vi "Initialize Signal Array.vi"(6 "error out":errorcluster, 9 "signal list":refnum<k21>[](array[refnum])) -> (0 "error out":errorcluster, 3 "Array":dbl[](array[numeric]))   [LabVIEW 2015]
uses:
  <vilib>/xnet/xnet.llb/XNET Database Open (Signal).vi
  <vilib>/xnet/xnet.llb/XNET Database Close (Signal).vi
  <resource>/objmgr/xnet.rc
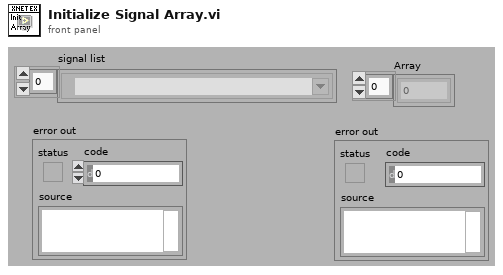
[diagram p1: front panel]
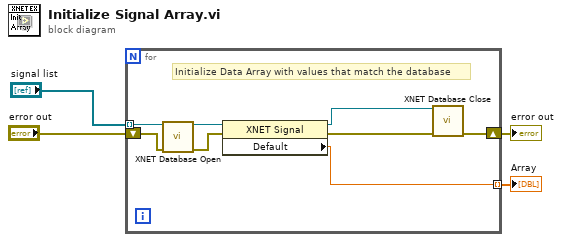
[diagram p0: block diagram]
diagram:
  n1 = for {
    tunnel: "signal list" -> [w12] mode=indexing
    shift-right: [w7] -> w3
    shift-left: "error out" -> [w11]
    tunnel: [w5] -> w1 mode=indexing
    # "Initialize Data Array with values that match the database"
    n2 = call-poly <vilib>:"XNET Database Open.vi"("signal in"=w12, "error in (no error)"=w11) -> ("signal out"=w10:refnum<k21>, "error out"=w9:errorcluster)  [unwired: 12 in]
    n3 = property class="XNET Signal"(reference=w10, error in=w9) -> (reference out=w6:refnum<k21>, error out=w8:errorcluster, "Default"=w5:dbl)
    n4 = call-poly <vilib>:"XNET Database Close.vi"("signal in"=w6, "error in (no error)"=w8) -> ("error out"=w7:errorcluster)  [unwired: 13 in]
  }
  "error out" <- w3
  "Array" <- w1
